vi "GatherTrunkVarsUnityControl.vi"() -> (12 "CenterPointForFF":dbl[](array[numeric]), 13 "Force Field Scaling Const K":dbl, 14 "FF Control Point":dbl[](array[numeric]), 15 "ForceZ and Moments":dbl[](array[numeric]), 16 "Radius":dbl, 17 "BoundaryYtrunk":dbl[](array[numeric]), 18 "BoundaryXtrunk":dbl[](array[numeric]), 19 "viconData":dbl[](array[numeric]))   [LabVIEW 2017]
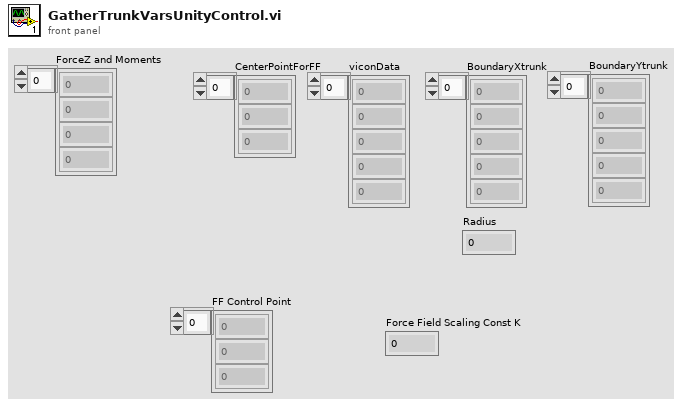
[diagram p1: front panel]
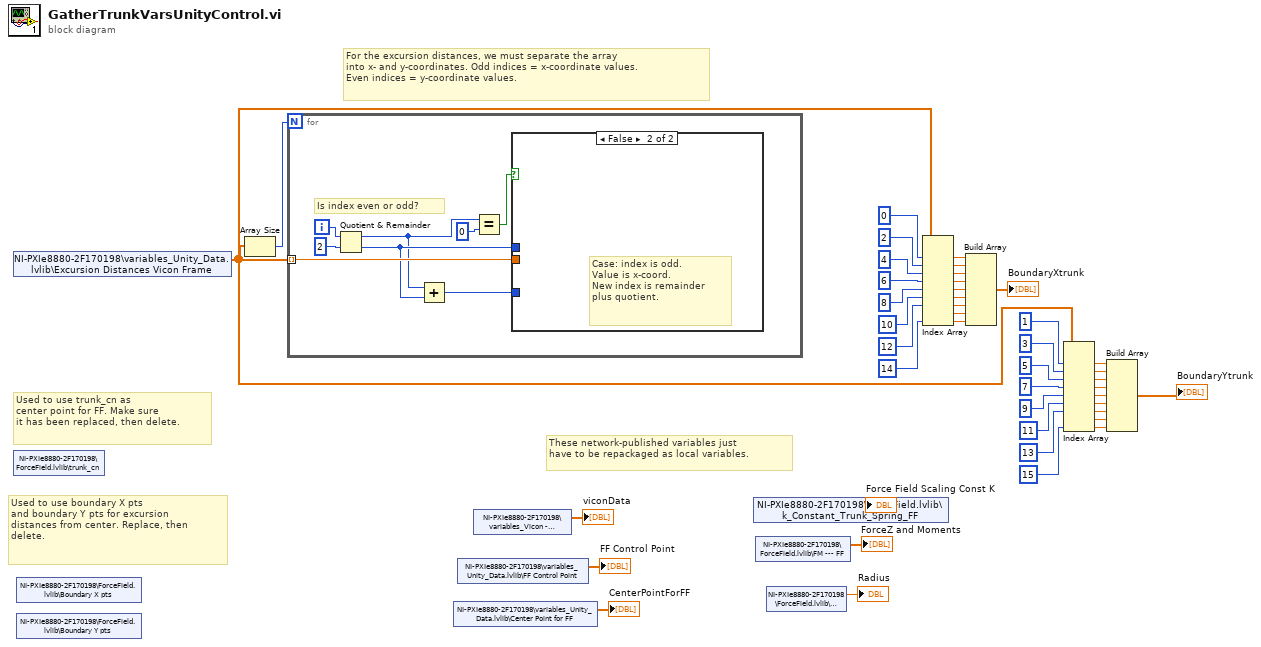
[diagram p0: block diagram]
diagram:
  # "These network-published variables just \nhave to be repackaged as local variables."
  # "Used to use boundary X pts\nand boundary Y pts for excursion \ndistances from center. Replace, then \ndelete."
  # "For the excursion distances, we must separate the array\ninto x- and y-coordinates. Odd indices = x-coordinate values. \nEven indices = y-coordinate values."
  # "Used to use trunk_cn as \ncenter point for FF. Make sure\nit has been replaced, then delete."
  n1 = shared-variable "NI-PXIe8880-2F170198\\variables_Unity_Data.lvlib\\Excursion Distances Vicon Frame"() -> (w2:dbl[])  [unwired: 1 in, 1 out]
  n2 = shared-variable "NI-PXIe8880-2F170198\\ForceField.lvlib\\trunk_cn"() -> ()  [unwired: 1 in, 2 out]
  n3 = shared-variable "NI-PXIe8880-2F170198\\ForceField.lvlib\\Boundary X pts"() -> ()  [unwired: 1 in, 2 out]
  n4 = shared-variable "NI-PXIe8880-2F170198\\ForceField.lvlib\\Boundary Y pts"() -> ()  [unwired: 1 in, 2 out]
  n5 = Array Size(array=w2) -> (size(s)=w38:i32)
  n6 = for {
    N: w38 -> [_]
    tunnel: w2 -> [w48] mode=indexing
    i -> [w52]
    # "Is index even or odd?"
    n7 = Quotient & Remainder(x=w52, y=2) -> (x-y*floor(x/y)=w46:i32, floor(x/y)=w47:i32)
    n8 = Add(x=w46, y=w47) -> (x+y=w45:i32)
    n9 = Equal?(x=w46, y=0) -> (x = y?=w49:bool)
    n10 = case shown="False" w49 {
      tunnel: w48 -> [_ _]
      tunnel: w47 -> [_ _]
      tunnel: w45 -> [_ _]
      frame True {
        # "Case: index is even.\nValue is y-coord. \nNew index is quotient."
      }
      frame False {
        # "Case: index is odd.\nValue is x-coord.\nNew index is remainder\nplus quotient."
      }
    }
  }
  n11 = shared-variable "NI-PXIe8880-2F170198\\variables_Unity_Data.lvlib\\Center Point for FF"() -> (→"CenterPointForFF":dbl[])  [unwired: 1 in, 1 out]
  n12 = shared-variable "NI-PXIe8880-2F170198\\variables_Unity_Data.lvlib\\FF Control Point"() -> (→"FF Control Point":dbl[])  [unwired: 1 in, 1 out]
  n13 = shared-variable "NI-PXIe8880-2F170198\\variables_Vicon - networkPublished.lvlib\\viconData"() -> (→"viconData":dbl[])  [unwired: 1 in, 1 out]
  n14 = shared-variable "NI-PXIe8880-2F170198\\ForceField.lvlib\\k_Constant_Trunk_Spring_FF"() -> (→"Force Field Scaling Const K":dbl)  [unwired: 1 in, 1 out]
  n15 = shared-variable "NI-PXIe8880-2F170198\\ForceField.lvlib\\FM --- FF"() -> (→"ForceZ and Moments":dbl[])  [unwired: 1 in, 1 out]
  n16 = shared-variable "NI-PXIe8880-2F170198\\ForceField.lvlib\\Radius"() -> (→"Radius":dbl)  [unwired: 1 in, 1 out]
  n17 = Index Array(array=w2, index #1=0 ("index"), index #2=2 ("index"), index #3=4 ("index"), index #4=6 ("index"), index #5=8 ("index"), index #6=10 ("index"), index #7=12 ("index"), index #9=14 ("index")) -> (element #1=w29:dbl, element #2=w28:dbl, element #3=w27:dbl, element #4=w26:dbl, element #5=w25:dbl, element #6=w24:dbl, element #7=w23:dbl, element #8=w22:dbl, element #9=w21:dbl)  [unwired: 1 in]
  n18 = Build Array(w29, w28, w27, w26, w25, w24, w23, w22, w21) -> (→"BoundaryXtrunk":dbl[])
  n19 = Index Array(array=w2, index #1=1 ("index"), index #2=3 ("index"), index #3=5 ("index"), index #4=7 ("index"), index #5=9 ("index"), index #6=11 ("index"), index #7=13 ("index"), index #9=15 ("index")) -> (element #1=w11:dbl, element #2=w10:dbl, element #3=w9:dbl, element #4=w8:dbl, element #5=w7:dbl, element #6=w6:dbl, element #7=w5:dbl, element #8=w4:dbl, element #9=w3:dbl)  [unwired: 1 in]
  n20 = Build Array(w11, w10, w9, w8, w7, w6, w5, w4, w3) -> (→"BoundaryYtrunk":dbl[])
